vi "AssetMgrGetMetricDefinitionsResponse_Parse.vi"(8 "error in (no error)":errorcluster, 11 "Message":T8) -> (0 "error out":errorcluster, 1 "Body":T1, 2 "Header":T7, 3 "AssetMgrGetMetricDefinitionsResponse":T6)   [LabVIEW 2017]
uses:
  <vilib>/addons/InsightCM/MessageBus/Base/controls/Message.ctl
  <vilib>/addons/InsightCM/MessageBus/Base/controls/MessageHeader.ctl
  <vilib>/addons/InsightCM/MessageBus/Base/controls/KeyValuePair.ctl
  <vilib>/addons/InsightCM/MessageBus/MessageLibrary/AssetManager/controls/AssetMgrGetMetricDefinitionsResponse.ctl
  <vilib>/addons/InsightCM/MessageBus/MessageLibrary/AssetManager/controls/AssetMgrGetMetricDefinitionsResponseBody.ctl
  <vilib>/addons/InsightCM/MessageBus/Base/controls/MetricDefinition.ctl
  <vilib>/addons/InsightCM/MessageBus/Base/controls/PropertyDefinition.ctl
  <vilib>/addons/InsightCM/MessageBus/Base/controls/ValidationRule.ctl
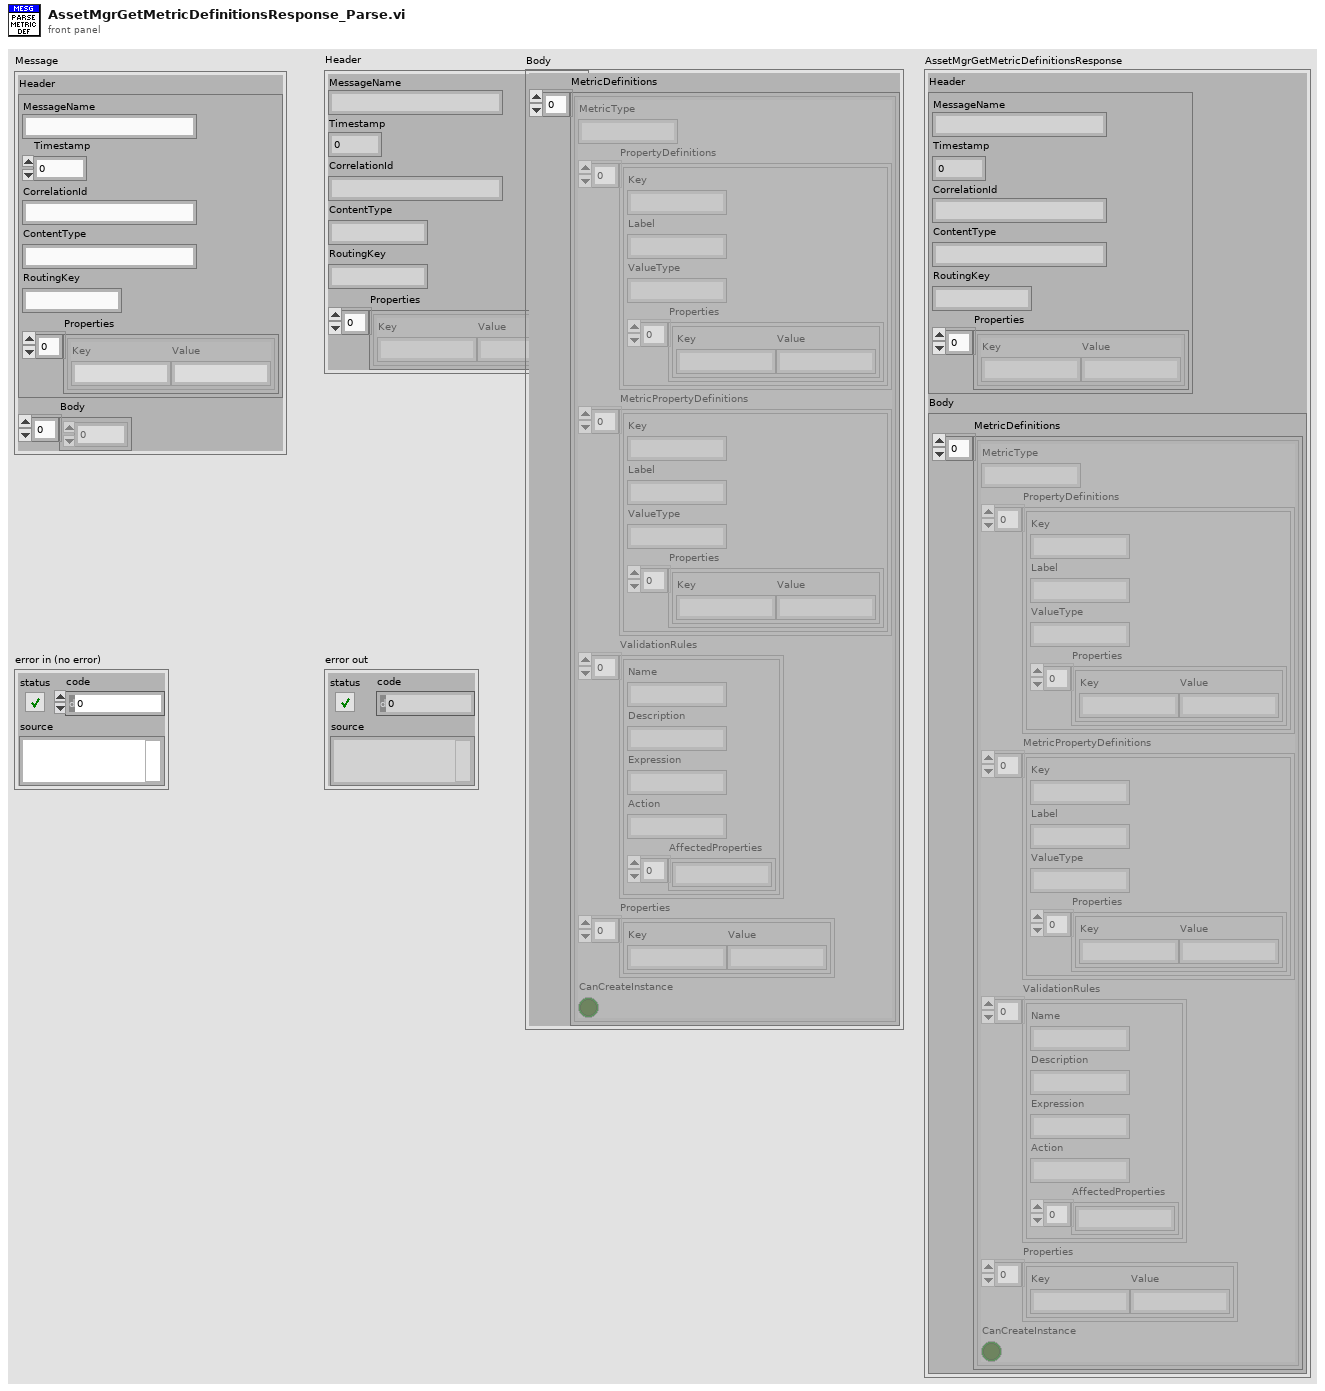
[diagram p1: front panel]
types:
  T1 = typedef "AssetMgrGetMetricDefinitionsResponseBody.ctl" = cluster{"MetricDefinitions":T2[]}
  T2 = typedef "MetricDefinition.ctl" = cluster{"MetricType":string, "PropertyDefinitions":T3[], "MetricPropertyDefinitions":T3[], "ValidationRules":T5[], "Properties":T4[], "CanCreateInstance":bool}
  T3 = typedef "PropertyDefinition.ctl" = cluster{"Key":string, "Label":string, "ValueType":string, "Properties":T4[]}
  T4 = typedef "KeyValuePair.ctl" = cluster{"Key":string, "Value":string}
  T5 = typedef "ValidationRule.ctl" = cluster{"Name":string, "Description":string, "Expression":string, "Action":string, "AffectedProperties":string[]}
  T6 = typedef "AssetMgrGetMetricDefinitionsResponse.ctl" = cluster{"Header":T7, "Body":T1}
  T7 = typedef "MessageHeader.ctl" = cluster{"MessageName":string, "Timestamp":i64, "CorrelationId":string, "ContentType":string, "RoutingKey":string, "Properties":T4[]}
  T8 = typedef "Message.ctl" = cluster{"Header":T7, "Body":u8[]}
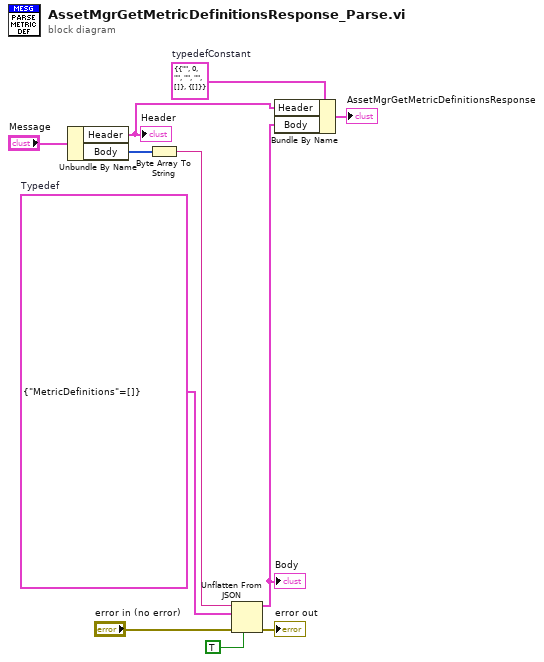
[diagram p0: block diagram]
diagram:
  w3 = T6 {"Header"={"MessageName"="", "Timestamp"=0, "CorrelationId"="", "ContentType"="", "RoutingKey"="", "Properties"=[]}, "Body"={"MetricDefinitions"=[]}}  # typedefConstant
  w7 = T1 {"MetricDefinitions"=[]}  # Typedef
  n1 = Unbundle By Name("Message") -> ("Header"=w9:T7, "Body"=w1:u8[])
  "Header" <- w9
  n2 = Byte Array To String(unsigned byte array=w1) -> (string=w6:string)
  n3 = Unflatten From JSON(JSON string=w6, type and defaults=w7, default null elements? (F)=TRUE, error in (no error)="error in (no error)") -> (value=w5:T1, error out=→"error out":errorcluster)  [unwired: 3 in]
  "Body" <- w5
  n4 = Bundle By Name(cluster=w3, "Header"=w9, "Body"=w5) -> (→"AssetMgrGetMetricDefinitionsResponse":T6)
